vi "Cambios de fase.vi"() -> ()   [LabVIEW 2021]
panel:
  out "Endotérmico":bool
  out "Exotérmico":bool
  in  "Proceso":dbl(ring) items=["Condensación", "Fusion ", "Sublimación", "Evaporación", "Deposición", "Solidificación"]
  out "Calor Latente":dbl(knob) scale=-1000.0..1000.0
  in  "stop":bool
  in  "Masa (g)":dbl caption="Masa"
  # "CAMBIOS DE FASE - AGUA"
  # "Calor Latente"
  # "kJ"
  # "gr"
  # "Desarrollado por:\n     Cesar Augusto Quiñones Segura\n     Andrea Carolina Sanchez Diaz\n     Jhon Erik Navarrete Gómez"
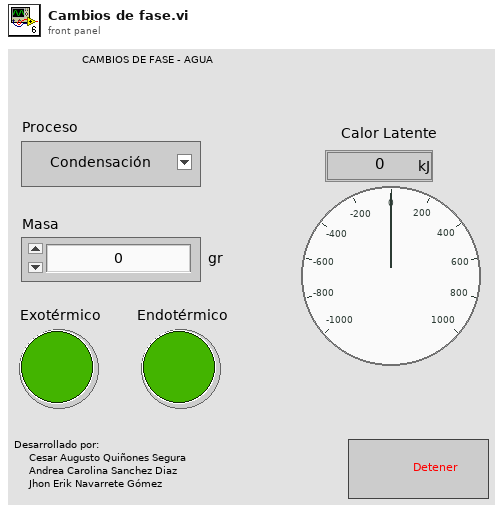
[diagram p1: front panel]
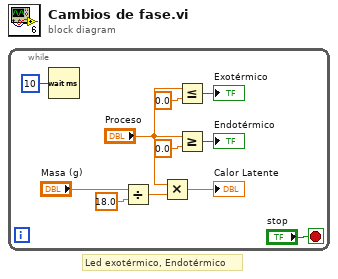
[diagram p0: block diagram]
diagram:
  # "Led exotérmico, Endotérmico"
  n1 = while {
    stop <- "stop" stop-if-true
    n2 = Wait (ms)(milliseconds to wait=u32 10) -> ()  [unwired: 1 out]
    n3 = Divide(x="Masa (g)", y=18.0) -> (x/y=w9:dbl)
    n4 = Multiply(x="Proceso", y=w9) -> (x*y=→"Calor Latente":dbl)
    n5 = Less Or Equal?(x="Proceso", y=0.0) -> (x <= y?=→"Exotérmico":bool)
    n6 = Greater Or Equal?(x="Proceso", y=0.0) -> (x >= y?=→"Endotérmico":bool)
  }
